vi "BRig_RT_panel_Laser2_v0,90.vi"(7 "input_setValues":bool, 9 "input_dataExp":u16[](array[numeric]), 11 "input_dataLC":u16[](array[numeric])) -> (1 "output_dataExp":u16[](array[numeric]), 3 "output_dataLC":u16[](array[numeric]))   [LabVIEW 2014]
panel:
  in  "LED_baseline":bool
  in  "Laser_power_step":dbl
  in  "Laser_power_max":dbl
  in  "Laser_power_min":dbl
  in  "Laser_Tshutter":u16=2
  in  "Laser_Freq":u16=10
  in  "Laser_Tpeak":u16=2
  in  "Laser_T":u16
  in  "LC_Sel_PostR_Count":u16
  in  "LC_Sel_PostR_Probability":u16
  in  "LC_Sel_PostR_Block":u16(slide) max=2 step=1 scale=0.0..2.0
  in  "LC_Sel_PostR_OnOff":bool
  in  "LC_Sel_PostR_Tdelay":u16
  in  "LC_Cue_PostR_Count":u16
  in  "LC_Cue_PostR_delayOpt":bool
  in  "LC_Cue_PostR_Probability":u16
  in  "LC_Cue_PostR_Block":u16(slide) max=2 step=1 scale=0.0..2.0
  in  "LC_Cue_PostR_OnOff":bool
  in  "LC_Cue_PostR_Tdelay":u16
  in  "LC_ENL_PostR_delayOpt":bool
  in  "LC_ENL_PostR_Count":u16
  in  "LC_ENL_PostR_Probability":u16 max=100 step=1
  in  "LC_ENL_PostR_Block":u16(slide) max=2 step=1 scale=0.0..2.0
  in  "LC_ENL_PostR_OnOff":bool
  in  "LC_ENL_PostR_Tdelay":u16
  in  "LC_Sel_PreR_Count":u16
  in  "LC_Sel_First_Count":u16
  in  "LC_Sel_PreR_Probability":u16
  in  "LC_Sel_PreR_Block":u16(slide) max=2 step=1 scale=0.0..2.0
  in  "LC_Sel_PreR_OnOff":bool
  in  "LC_Sel_First_Probability":u16
  in  "LC_Sel_First_Block":u16(slide) max=2 step=1 scale=0.0..2.0
  in  "LC_Sel_First_OnOff":bool
  in  "LC_Sel_PreR_Tdelay":u16
  in  "LC_Sel_First_Tdelay":u16
  in  "LC_Cue_PreR_Count":u16
  in  "LC_Cue_First_Count":u16
  in  "LC_Cue_PreR_delayOpt":bool
  in  "LC_ENL_PreR_delayOpt":bool
  in  "LC_ENL_PreR_Count":u16
  in  "LC_ENL_First_Count":u16
  in  "LC_Cue_First_delayOpt":bool
  in  "LC_ENL_First_delayOpt":bool
  in  "LC_Wrong_Probability":u16
  in  "LC_Wrong_Trial":u16(slide) max=2 step=1 scale=0.0..2.0
  in  "LC_Wrong_Block":u16(slide) max=2 step=1 scale=0.0..2.0
  in  "LC_Wrong_OnOff":bool
  in  "LC_Reward_Probability":u16
  in  "LC_Reward_Trial":u16(slide) max=2 step=1 scale=0.0..2.0
  in  "LC_Reward_Block":u16(slide) max=2 step=1 scale=0.0..2.0
  in  "LC_Reward_OnOff":bool
  in  "LC_Cue_PreR_Probability":u16
  in  "LC_Cue_PreR_Block":u16(slide) max=2 step=1 scale=0.0..2.0
  in  "LC_Cue_PreR_OnOff":bool
  in  "LC_Cue_First_Probability":u16
  in  "LC_Cue_First_Block":u16(slide) max=2 step=1 scale=0.0..2.0
  in  "LC_Cue_First_OnOff":bool
  in  "LC_ENL_PreR_Probability":u16 max=100 step=1
  in  "LC_ENL_PreR_Block":u16(slide) max=2 step=1 scale=0.0..2.0
  in  "LC_ENL_PreR_OnOff":bool
  in  "LC_ENL_First_Probability":u16 max=100 step=1
  in  "LC_ENL_First_Block":u16(slide) max=2 step=1 scale=0.0..2.0
  in  "LC_Wrong_Tdelay":u16
  in  "LC_Cue_PreR_Tdelay":u16
  in  "LC_ENL_PreR_Tdelay":u16
  in  "LC_Reward_Tdelay":u16
  in  "LC_Cue_First_Tdelay":u16
  in  "LC_ENL_First_Tdelay":u16
  in  "LC_ENL_First_OnOff":bool
  # "Laser2 Control\n                               On/Off      Block        Probability [%]   Delay [ms]                              Count"
  # "Enforced\nNonLick"
  # "from end"
  # "First\nTrial"
  # "from start"
  # "from end"
  # "PreReward\nTrials"
  # "from start"
  # "from end"
  # "PostReward\nTrials"
  # "from start"
  # "Cue"
  # "from end"
  # "First\nTrial"
  # "from start"
  # "from end"
  # "PreReward\nTrials"
  # "from start"
  # "from end"
  # "PreReward\nTrials"
  # "from start"
  # "Selection"
  # "from start"
  # "First\nTrial"
  # "from start"
  # "PreReward\nTrials"
  # "from start"
  # "PostReward\nTrials"
  # "Laser2 Parameters"
  # "Laser2 Response\n           On/Off      Block           Trial     Probability %  Delay [ms]"
  # "Frequency\n[Hz]"
  # "Selection\nReward"
  # "Timing [ms]\n Duration     Peak Width   Shutter"
  # "Selection\nWrong"
  # "Laser Power [V]\nMin          Max              Step"
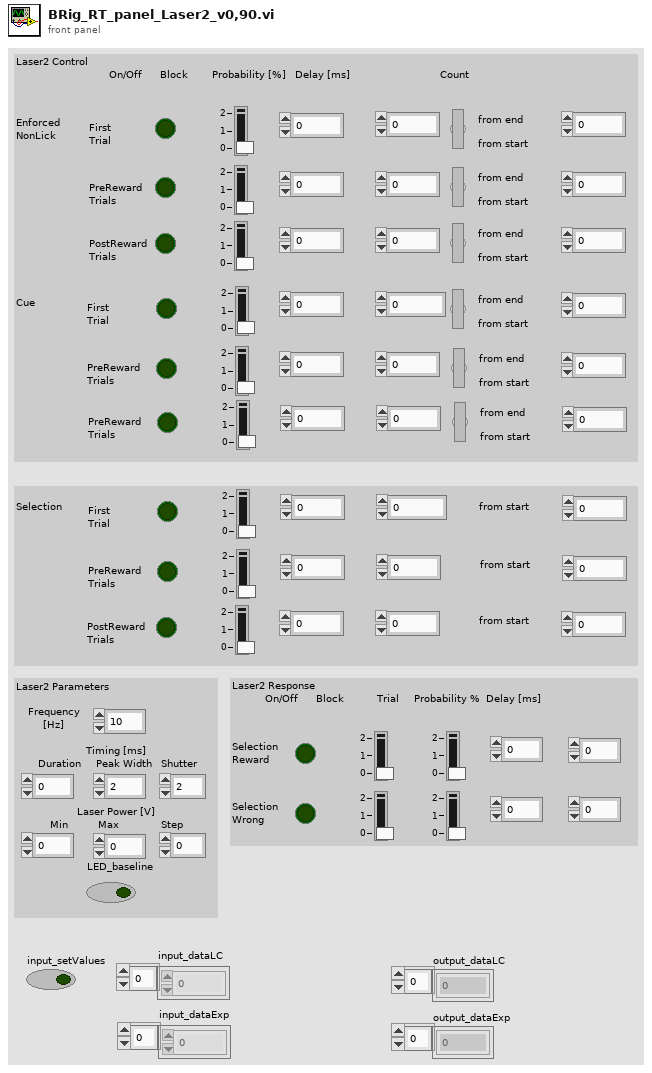
[diagram p1: front panel]
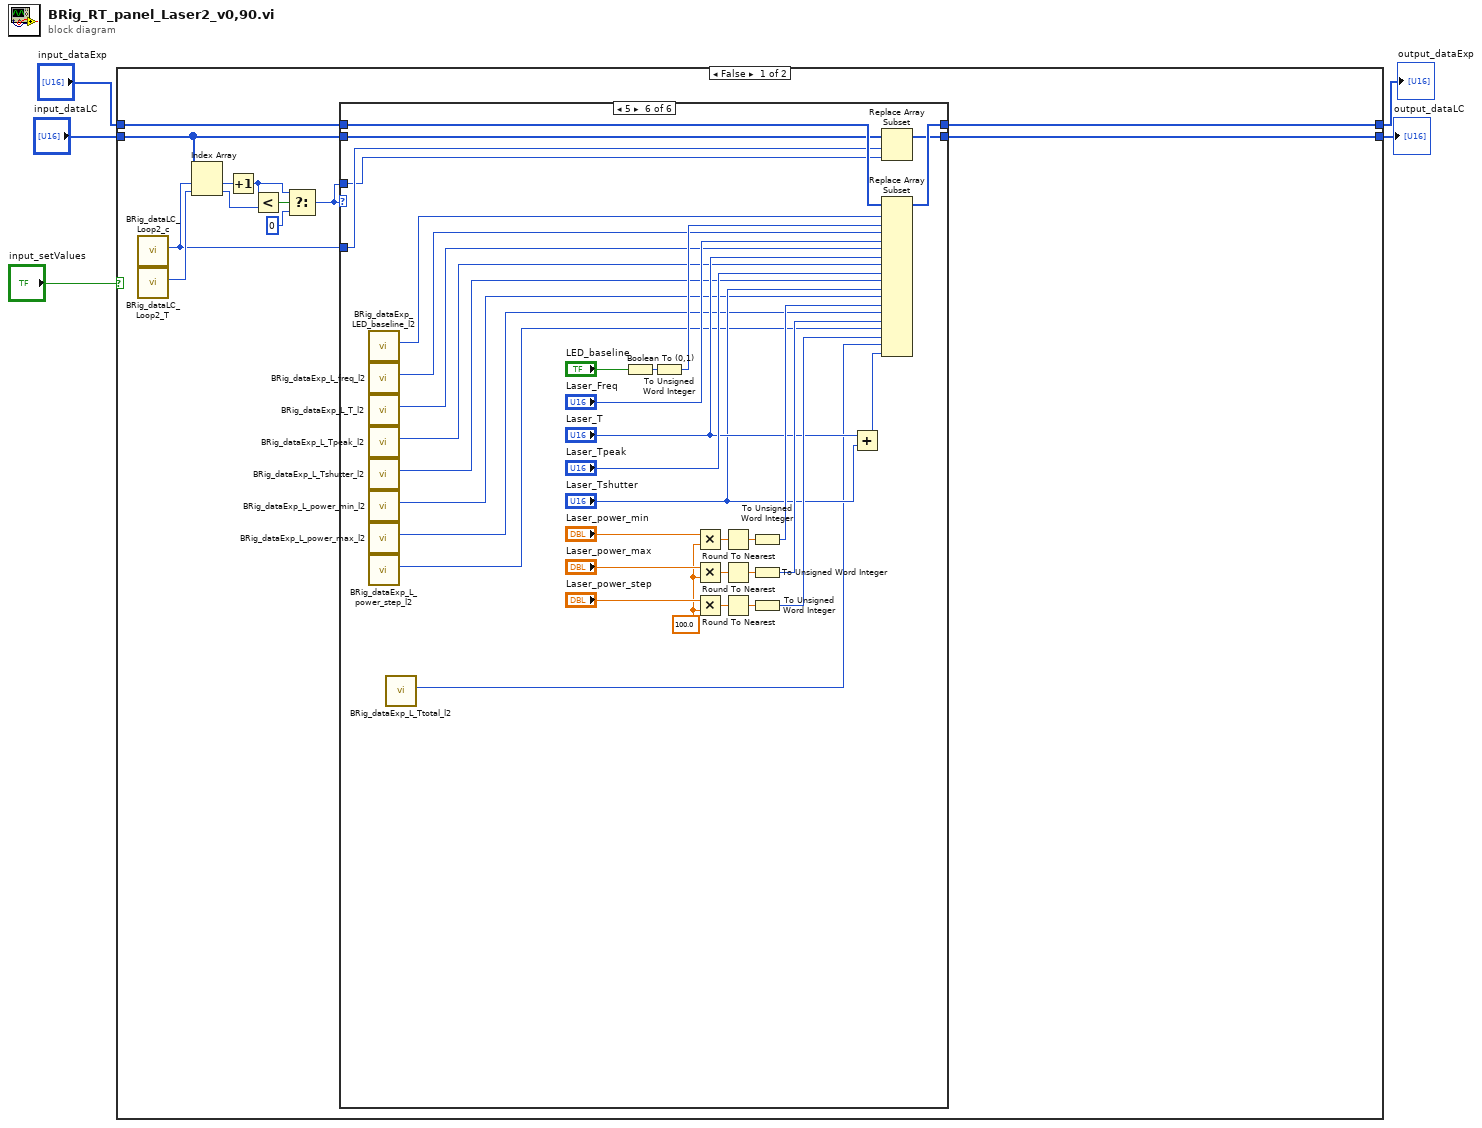
[diagram p0: block diagram]
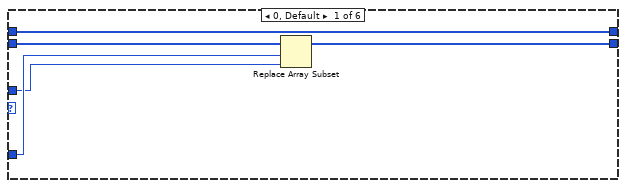
[diagram p2: hidden frame]
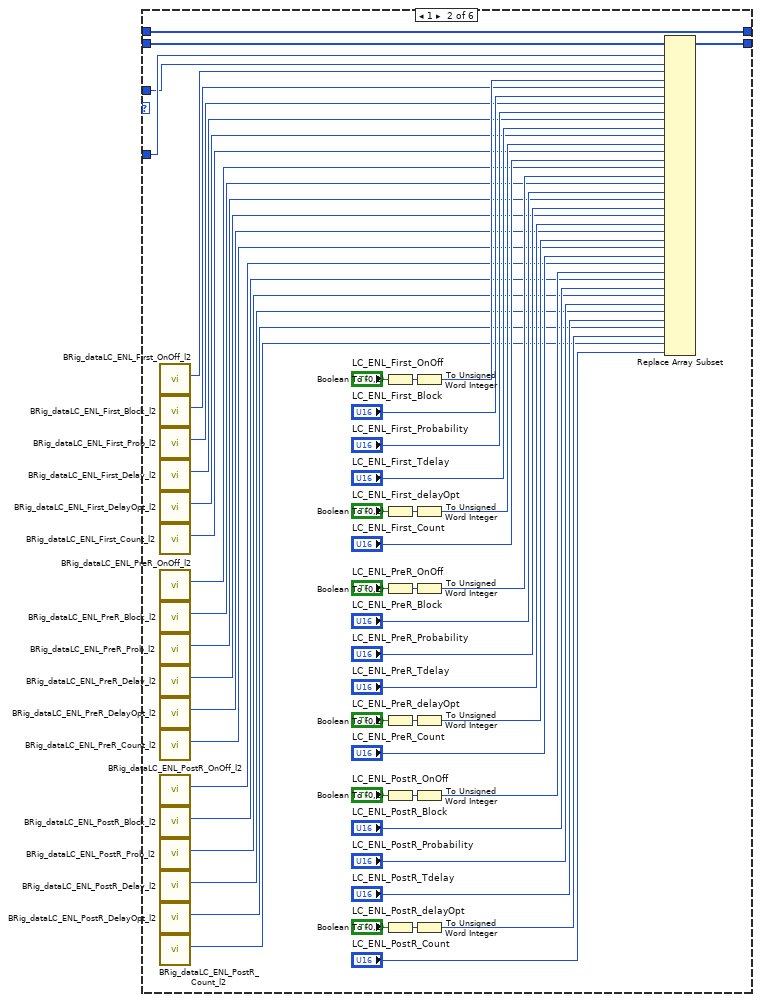
[diagram p3: hidden frame]
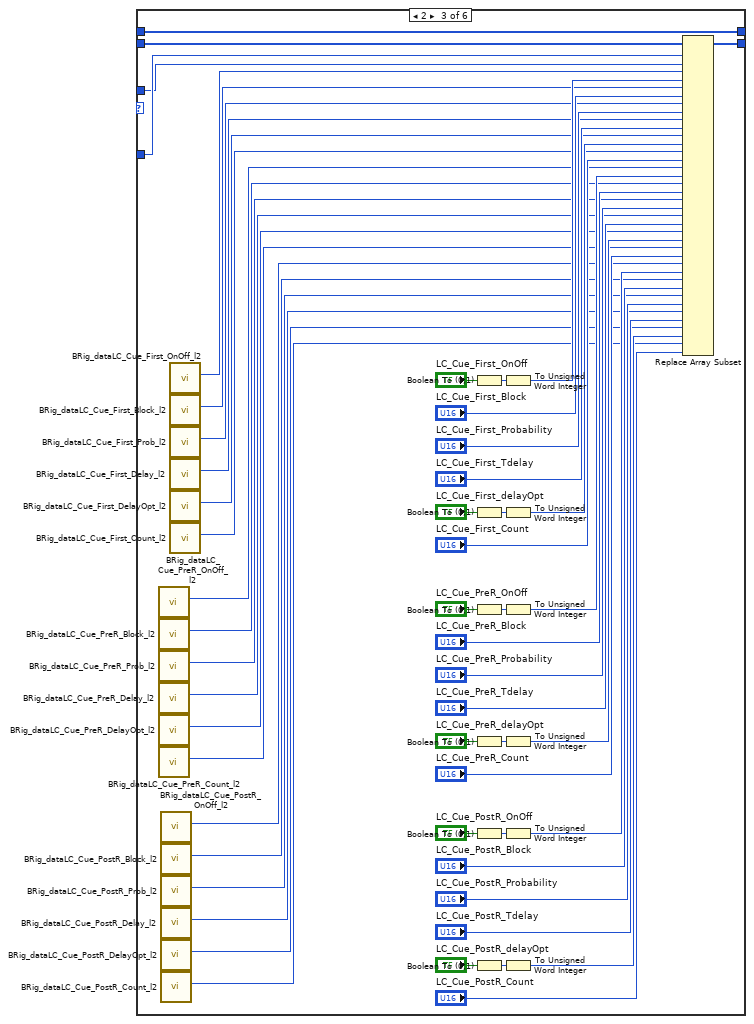
[diagram p4: hidden frame]
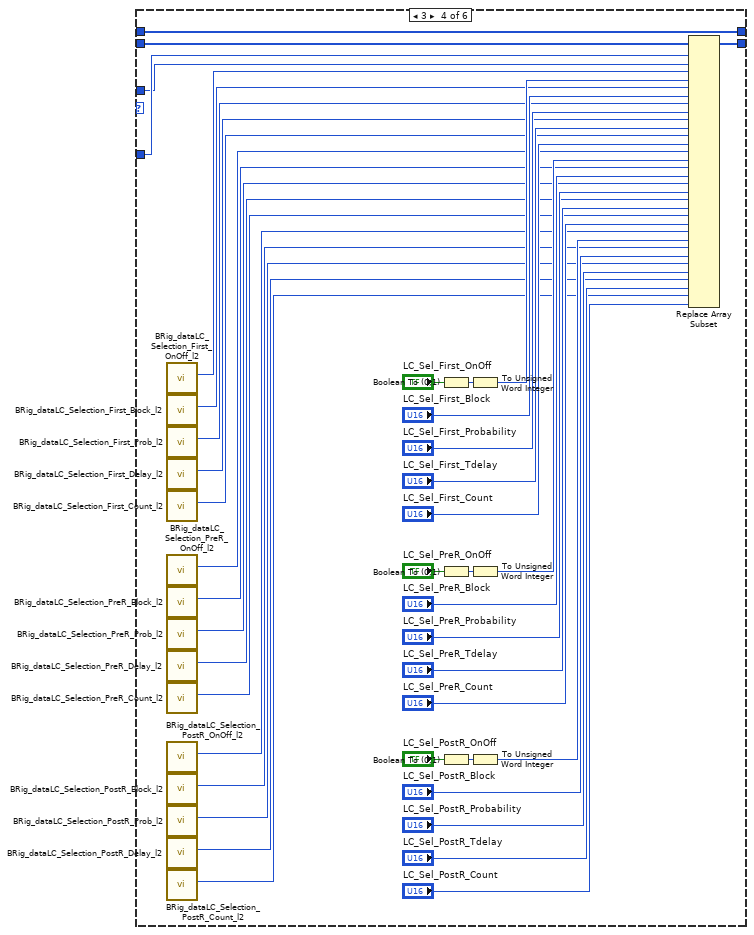
[diagram p5: hidden frame]
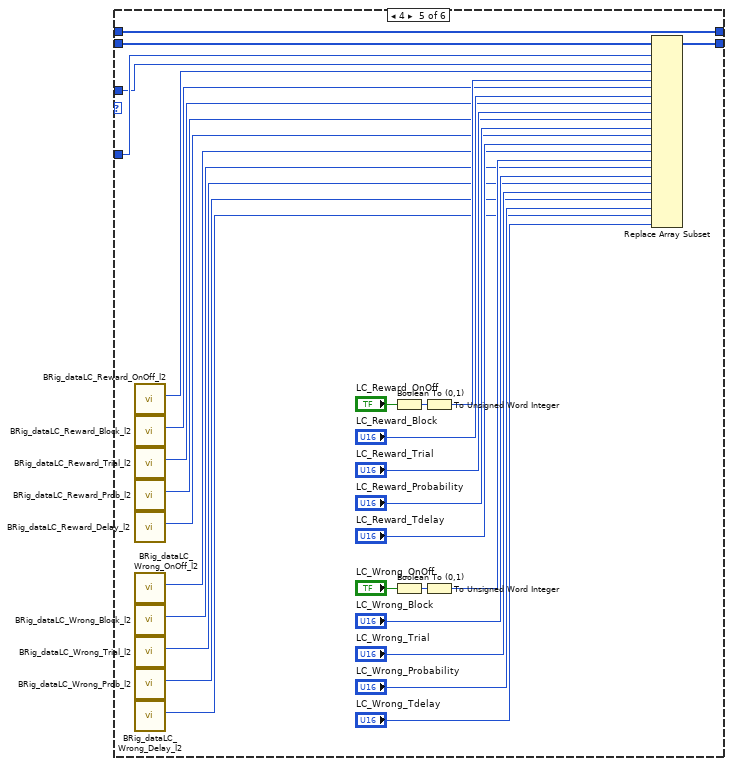
[diagram p6: hidden frame]
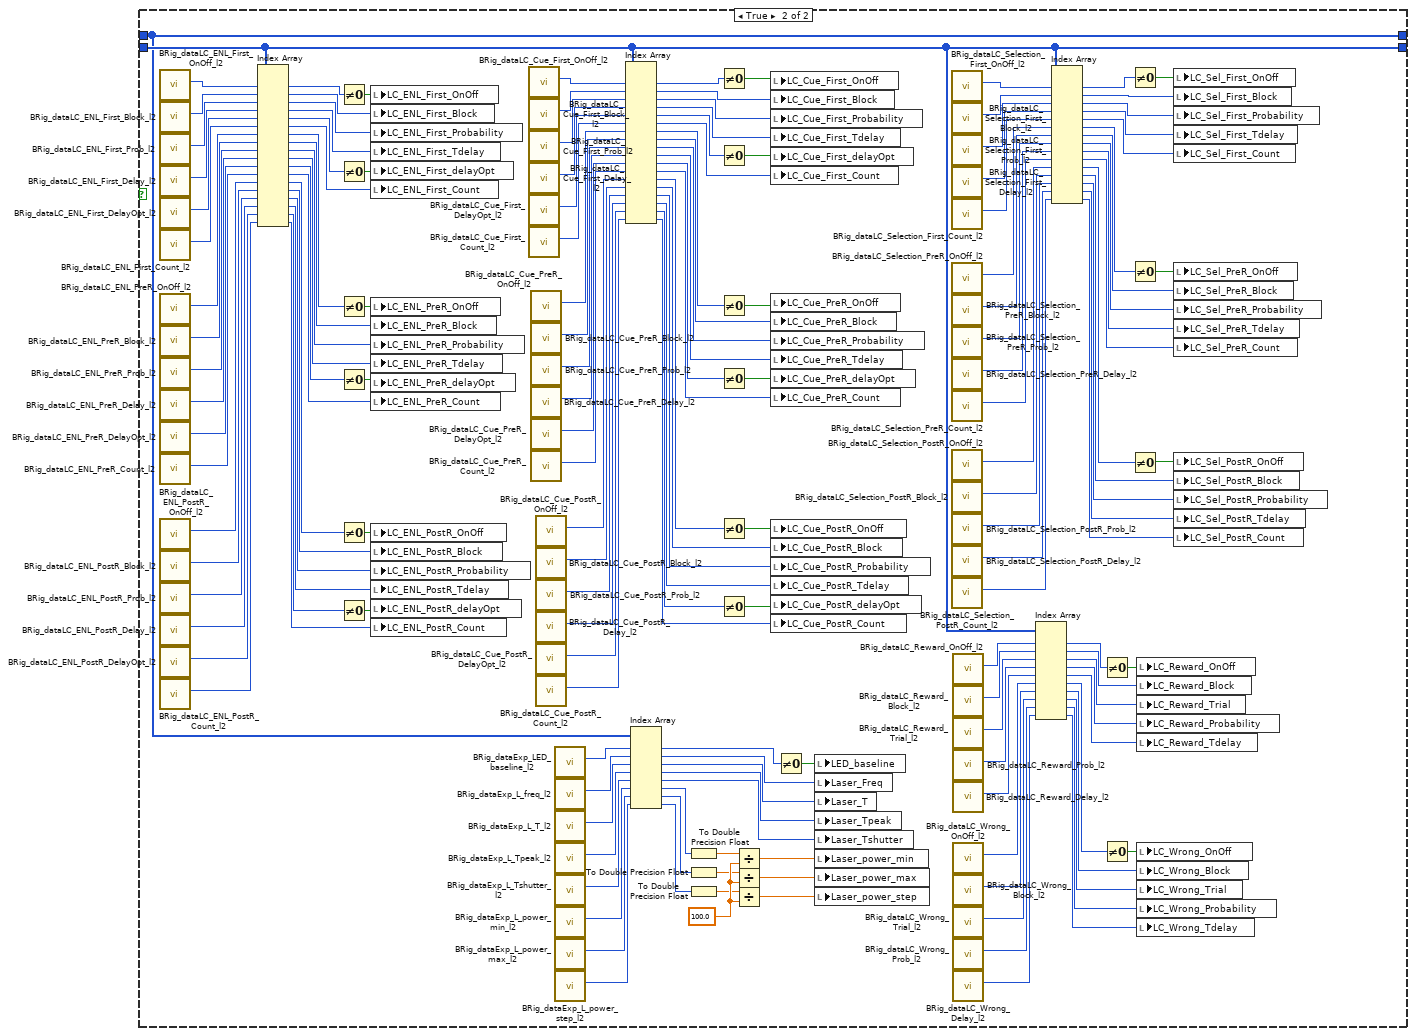
[diagram p7: hidden frame]
diagram:
  n1 = case shown="False" "input_setValues" {
    tunnel: "input_dataLC" -> [w17 w321]
    tunnel: [w11 w321] -> w4
    tunnel: "input_dataExp" -> [w7 w235]
    tunnel: [w6 w235] -> w1
    frame False {
      n2 = call "BRig_dataLC_Loop2_c.vi"() -> ("output_Loop2_c"=w8:i32)  [unwired: 11 in]
      n3 = call "BRig_dataLC_Loop2_T.vi"() -> ("output_Loop2_T"=w9:i32)  [unwired: 11 in]
      n4 = Index Array(array=w17, index #1=w8, index #2=w9) -> (element #1=w16:u16, element #2=w15:u16)
      n5 = Increment(x=w16) -> (x+1=w12:u16)
      n6 = Less?(x=w12, y=w15) -> (x < y?=w14:bool)
      n7 = Select(t=w12, s=w14, f=u16 0) -> (s? t:f=w10:u16)
      n8 = case shown="5" w10 {
        tunnel: w17 -> [w22 w75 w128 w169 w198 w202]
        tunnel: w8 -> [w20 w43 w96 w146 w182 w200]
        tunnel: w10 -> [w19 w42 w95 w145 w181 w199]
        tunnel: [w21 w74 w127 w168 w197 w201] -> w11
        tunnel: w7 -> [w18 w23 w76 w129 w170 w204]
        tunnel: [w18 w23 w76 w129 w170 w203] -> w6
        frame 0, Default {
          n9 = Replace Array Subset(array=w22, new element=w19, index=w20) -> (w21:u16[])
        }
        frame 1 {
          n10 = call "BRig_dataLC_ENL_First_OnOff_l2.vi"() -> ("output_ENL_First_OnOff_l2"=w24:i32)  [unwired: 11 in]
          n11 = call "BRig_dataLC_ENL_First_Block_l2.vi"() -> ("output_ENL_First_Block_l2"=w25:i32)  [unwired: 11 in]
          n12 = call "BRig_dataLC_ENL_First_Prob_l2.vi"() -> ("output_ENL_First_Prob_l2"=w26:i32)  [unwired: 11 in]
          n13 = call "BRig_dataLC_ENL_First_Delay_l2.vi"() -> ("output_ENL_First_Delay_l2"=w27:i32)  [unwired: 11 in]
          n14 = call "BRig_dataLC_ENL_First_DelayOpt_l2.vi"() -> ("output_ENL_First_DelayOpt_l2"=w28:i32)  [unwired: 11 in]
          n15 = call "BRig_dataLC_ENL_First_Count_l2.vi"() -> ("output_ENL_First_Count_l2"=w39:i32)  [unwired: 11 in]
          n16 = call "BRig_dataLC_ENL_PreR_OnOff_l2.vi"() -> ("output_ENL_PreR_OnOff_l2"=w29:i32)  [unwired: 11 in]
          n17 = call "BRig_dataLC_ENL_PreR_Block_l2.vi"() -> ("output_ENL_PreR_Block_l2"=w31:i32)  [unwired: 11 in]
          n18 = call "BRig_dataLC_ENL_PreR_Prob_l2.vi"() -> ("output_ENL_PreR_Prob_l2"=w30:i32)  [unwired: 11 in]
          n19 = call "BRig_dataLC_ENL_PreR_Delay_l2.vi"() -> ("output_ENL_PreR_Delay_l2"=w32:i32)  [unwired: 11 in]
          n20 = call "BRig_dataLC_ENL_PreR_DelayOpt_l2.vi"() -> ("output_ENL_PreR_DelayOpt_l2"=w33:i32)  [unwired: 11 in]
          n21 = call "BRig_dataLC_ENL_PreR_Count_l2.vi"() -> ("output_ENL_PreR_Count_l2"=w40:i32)  [unwired: 11 in]
          n22 = call "BRig_dataLC_ENL_PostR_OnOff_l2.vi"() -> ("output_ENL_PostR_OnOff_l2"=w34:i32)  [unwired: 11 in]
          n23 = call "BRig_dataLC_ENL_PostR_Block_l2.vi"() -> ("output_ENL_PostR_Block_l2"=w35:i32)  [unwired: 11 in]
          n24 = call "BRig_dataLC_ENL_PostR_Prob_l2.vi"() -> ("output_ENL_PostR_Prob_l2"=w36:i32)  [unwired: 11 in]
          n25 = call "BRig_dataLC_ENL_PostR_Delay_l2.vi"() -> ("output_ENL_PostR_Delay_l2"=w37:i32)  [unwired: 11 in]
          n26 = call "BRig_dataLC_ENL_PostR_DelayOpt_l2.vi"() -> ("output_ENL_PostR_DelayOpt_l2"=w38:i32)  [unwired: 11 in]
          n27 = call "BRig_dataLC_ENL_PostR_Count_l2.vi"() -> ("output_ENL_PostR_Count_l2"=w41:i32)  [unwired: 11 in]
          n28 = Boolean To (0,1)(Boolean="LC_ENL_First_OnOff") -> (0, 1=w72:i16)
          n29 = Boolean To (0,1)(Boolean="LC_ENL_First_delayOpt") -> (0, 1=w71:i16)
          n30 = Boolean To (0,1)(Boolean="LC_ENL_PreR_OnOff") -> (0, 1=w69:i16)
          n31 = Boolean To (0,1)(Boolean="LC_ENL_PreR_delayOpt") -> (0, 1=w67:i16)
          n32 = Boolean To (0,1)(Boolean="LC_ENL_PostR_OnOff") -> (0, 1=w65:i16)
          n33 = Boolean To (0,1)(Boolean="LC_ENL_PostR_delayOpt") -> (0, 1=w63:i16)
          n34 = To Unsigned Word Integer(number=w72) -> (unsigned 16bit integer=w61:u16)
          n35 = To Unsigned Word Integer(number=w71) -> (unsigned 16bit integer=w57:u16)
          n36 = To Unsigned Word Integer(number=w69) -> (unsigned 16bit integer=w55:u16)
          n37 = To Unsigned Word Integer(number=w67) -> (unsigned 16bit integer=w51:u16)
          n38 = To Unsigned Word Integer(number=w65) -> (unsigned 16bit integer=w49:u16)
          n39 = To Unsigned Word Integer(number=w63) -> (unsigned 16bit integer=w45:u16)
          n40 = Replace Array Subset(array=w75, new element #1=w42, index #1=w43, new element #2=w61, index #2=w24, new element #3="LC_ENL_First_Block", index #3=w25, new element #4="LC_ENL_First_Probability", index #4=w26, new element #5="LC_ENL_First_Tdelay", index #5=w27, new element #6=w57, index #6=w28, new element #7="LC_ENL_First_Count", index #7=w39, new element #8=w55, index #8=w29, new element #9="LC_ENL_PreR_Block", index #9=w31, new element #10="LC_ENL_PreR_Probability", index #10=w30, new element #11="LC_ENL_PreR_Tdelay", index #11=w32, new element #12=w51, index #12=w33, new element #13="LC_ENL_PreR_Count", index #13=w40, new element #14=w49, index #14=w34, new element #15="LC_ENL_PostR_Block", index #15=w35, new element #16="LC_ENL_PostR_Probability", index #16=w36, new element #17="LC_ENL_PostR_Tdelay", index #17=w37, new element #18=w45, index #18=w38, new element #19="LC_ENL_PostR_Count", index #19=w41) -> (w74:u16[])
        }
        frame 2 {
          n41 = call "BRig_dataLC_Cue_PreR_OnOff_l2.vi"() -> ("output_Cue_PreR_OnOff_l2"=w83:i32)  [unwired: 11 in]
          n42 = call "BRig_dataLC_Cue_PreR_Block_l2.vi"() -> ("output_Cue_PreR_Block_l2"=w84:i32)  [unwired: 11 in]
          n43 = call "BRig_dataLC_Cue_PreR_Prob_l2.vi"() -> ("output_Cue_PreR_Prob_l2"=w85:i32)  [unwired: 11 in]
          n44 = call "BRig_dataLC_Cue_PreR_Delay_l2.vi"() -> ("output_Cue_PreR_Delay_l2"=w86:i32)  [unwired: 11 in]
          n45 = call "BRig_dataLC_Cue_PreR_DelayOpt_l2.vi"() -> ("output_Cue_PreR_DelayOpt_l2"=w87:i32)  [unwired: 11 in]
          n46 = call "BRig_dataLC_Cue_PreR_Count_l2.vi"() -> ("output_Cue_PreR_Count_l2"=w88:i32)  [unwired: 11 in]
          n47 = call "BRig_dataLC_Cue_PostR_OnOff_l2.vi"() -> ("output_Cue_PostR_OnOff_l2"=w82:i32)  [unwired: 11 in]
          n48 = call "BRig_dataLC_Cue_PostR_Block_l2.vi"() -> ("output_Cue_PostR_Block_l2"=w77:i32)  [unwired: 11 in]
          n49 = call "BRig_dataLC_Cue_PostR_Prob_l2.vi"() -> ("output_Cue_PostR_Prob_l2"=w78:i32)  [unwired: 11 in]
          n50 = call "BRig_dataLC_Cue_PostR_Delay_l2.vi"() -> ("output_Cue_PostR_Delay_l2"=w79:i32)  [unwired: 11 in]
          n51 = call "BRig_dataLC_Cue_PostR_DelayOpt_l2.vi"() -> ("output_Cue_PostR_DelayOpt_l2"=w80:i32)  [unwired: 11 in]
          n52 = call "BRig_dataLC_Cue_PostR_Count_l2.vi"() -> ("output_Cue_PostR_Count_l2"=w81:i32)  [unwired: 11 in]
          n53 = call "BRig_dataLC_Cue_First_OnOff_l2.vi"() -> ("output_Cue_First_OnOff_l2"=w89:i32)  [unwired: 11 in]
          n54 = call "BRig_dataLC_Cue_First_Block_l2.vi"() -> ("output_Cue_First_Block_l2"=w90:i32)  [unwired: 11 in]
          n55 = call "BRig_dataLC_Cue_First_Prob_l2.vi"() -> ("output_Cue_First_Prob_l2"=w91:i32)  [unwired: 11 in]
          n56 = call "BRig_dataLC_Cue_First_Delay_l2.vi"() -> ("output_Cue_First_Delay_l2"=w92:i32)  [unwired: 11 in]
          n57 = call "BRig_dataLC_Cue_First_DelayOpt_l2.vi"() -> ("output_Cue_First_DelayOpt_l2"=w93:i32)  [unwired: 11 in]
          n58 = call "BRig_dataLC_Cue_First_Count_l2.vi"() -> ("output_Cue_First_Count_l2"=w94:i32)  [unwired: 11 in]
          n59 = Boolean To (0,1)(Boolean="LC_Cue_First_OnOff") -> (0, 1=w120:i16)
          n60 = Boolean To (0,1)(Boolean="LC_Cue_First_delayOpt") -> (0, 1=w119:i16)
          n61 = Boolean To (0,1)(Boolean="LC_Cue_PreR_OnOff") -> (0, 1=w118:i16)
          n62 = Boolean To (0,1)(Boolean="LC_Cue_PreR_delayOpt") -> (0, 1=w117:i16)
          n63 = Boolean To (0,1)(Boolean="LC_Cue_PostR_OnOff") -> (0, 1=w116:i16)
          n64 = Boolean To (0,1)(Boolean="LC_Cue_PostR_delayOpt") -> (0, 1=w115:i16)
          n65 = To Unsigned Word Integer(number=w120) -> (unsigned 16bit integer=w114:u16)
          n66 = To Unsigned Word Integer(number=w119) -> (unsigned 16bit integer=w110:u16)
          n67 = To Unsigned Word Integer(number=w118) -> (unsigned 16bit integer=w108:u16)
          n68 = To Unsigned Word Integer(number=w117) -> (unsigned 16bit integer=w104:u16)
          n69 = To Unsigned Word Integer(number=w116) -> (unsigned 16bit integer=w102:u16)
          n70 = To Unsigned Word Integer(number=w115) -> (unsigned 16bit integer=w98:u16)
          n71 = Replace Array Subset(array=w128, new element #1=w95, index #1=w96, new element #2=w114, index #2=w89, new element #3="LC_Cue_First_Block", index #3=w90, new element #4="LC_Cue_First_Probability", index #4=w91, new element #5="LC_Cue_First_Tdelay", index #5=w92, new element #6=w110, index #6=w93, new element #7="LC_Cue_First_Count", index #7=w94, new element #8=w108, index #8=w83, new element #9="LC_Cue_PreR_Block", index #9=w84, new element #10="LC_Cue_PreR_Probability", index #10=w85, new element #11="LC_Cue_PreR_Tdelay", index #11=w86, new element #12=w104, index #12=w87, new element #13="LC_Cue_PreR_Count", index #13=w88, new element #14=w102, index #14=w82, new element #15="LC_Cue_PostR_Block", index #15=w77, new element #16="LC_Cue_PostR_Probability", index #16=w78, new element #17="LC_Cue_PostR_Tdelay", index #17=w79, new element #18=w98, index #18=w80, new element #19="LC_Cue_PostR_Count", index #19=w81) -> (w127:u16[])
        }
        frame 3 {
          n72 = call "BRig_dataLC_Selection_First_OnOff_l2.vi"() -> ("output_Selection_First_OnOff_l2"=w130:i32)  [unwired: 11 in]
          n73 = call "BRig_dataLC_Selection_First_Block_l2.vi"() -> ("output_Selection_First_Block_l2"=w131:i32)  [unwired: 11 in]
          n74 = call "BRig_dataLC_Selection_First_Prob_l2.vi"() -> ("output_Selection_First_Prob_l2"=w132:i32)  [unwired: 11 in]
          n75 = call "BRig_dataLC_Selection_First_Delay_l2.vi"() -> ("output_Selection_First_Delay_l2"=w133:i32)  [unwired: 11 in]
          n76 = call "BRig_dataLC_Selection_First_Count_l2.vi"() -> ("output_Selection_First_Count_l2"=w134:i32)  [unwired: 11 in]
          n77 = call "BRig_dataLC_Selection_PreR_OnOff_l2.vi"() -> ("output_Selection_PreR_OnOff_l2"=w135:i32)  [unwired: 11 in]
          n78 = call "BRig_dataLC_Selection_PreR_Block_l2.vi"() -> ("output_Selection_PreR_Block_l2"=w136:i32)  [unwired: 11 in]
          n79 = call "BRig_dataLC_Selection_PreR_Prob_l2.vi"() -> ("output_Selection_PreR_Prob_l2"=w137:i32)  [unwired: 11 in]
          n80 = call "BRig_dataLC_Selection_PreR_Delay_l2.vi"() -> ("output_Selection_PreR_Delay_l2"=w138:i32)  [unwired: 11 in]
          n81 = call "BRig_dataLC_Selection_PreR_Count_l2.vi"() -> ("output_Selection_PreR_Count_l2"=w139:i32)  [unwired: 11 in]
          n82 = call "BRig_dataLC_Selection_PostR_OnOff_l2.vi"() -> ("output_Selection_PostR_OnOff_l2"=w140:i32)  [unwired: 11 in]
          n83 = call "BRig_dataLC_Selection_PostR_Block_l2.vi"() -> ("output_Selection_PostR_Block_l2"=w141:i32)  [unwired: 11 in]
          n84 = call "BRig_dataLC_Selection_PostR_Prob_l2.vi"() -> ("output_Selection_PostR_Prob_l2"=w142:i32)  [unwired: 11 in]
          n85 = call "BRig_dataLC_Selection_PostR_Delay_l2.vi"() -> ("output_Selection_PostR_Delay_l2"=w143:i32)  [unwired: 11 in]
          n86 = call "BRig_dataLC_Selection_PostR_Count_l2.vi"() -> ("output_Selection_PostR_Count_l2"=w144:i32)  [unwired: 11 in]
          n87 = Boolean To (0,1)(Boolean="LC_Sel_First_OnOff") -> (0, 1=w164:i16)
          n88 = Boolean To (0,1)(Boolean="LC_Sel_PreR_OnOff") -> (0, 1=w163:i16)
          n89 = Boolean To (0,1)(Boolean="LC_Sel_PostR_OnOff") -> (0, 1=w162:i16)
          n90 = To Unsigned Word Integer(number=w164) -> (unsigned 16bit integer=w161:u16)
          n91 = To Unsigned Word Integer(number=w163) -> (unsigned 16bit integer=w156:u16)
          n92 = To Unsigned Word Integer(number=w162) -> (unsigned 16bit integer=w151:u16)
          n93 = Replace Array Subset(array=w169, new element #1=w145, index #1=w146, new element #2=w161, index #2=w130, new element #3="LC_Sel_First_Block", index #3=w131, new element #4="LC_Sel_First_Probability", index #4=w132, new element #5="LC_Sel_First_Tdelay", index #5=w133, new element #6="LC_Sel_First_Count", index #6=w134, new element #7=w156, index #7=w135, new element #8="LC_Sel_PreR_Block", index #8=w136, new element #9="LC_Sel_PreR_Probability", index #9=w137, new element #10="LC_Sel_PreR_Tdelay", index #10=w138, new element #11="LC_Sel_PreR_Count", index #11=w139, new element #12=w151, index #12=w140, new element #13="LC_Sel_PostR_Block", index #13=w141, new element #14="LC_Sel_PostR_Probability", index #14=w142, new element #15="LC_Sel_PostR_Tdelay", index #15=w143, new element #16="LC_Sel_PostR_Count", index #16=w144) -> (w168:u16[])
        }
        frame 4 {
          n94 = call "BRig_dataLC_Reward_OnOff_l2.vi"() -> ("output_Reward_OnOff_l2"=w171:i32)  [unwired: 11 in]
          n95 = call "BRig_dataLC_Reward_Block_l2.vi"() -> ("output_Reward_Block_l2"=w172:i32)  [unwired: 11 in]
          n96 = call "BRig_dataLC_Reward_Trial_l2.vi"() -> ("output_Reward_Trial_l2"=w173:i32)  [unwired: 11 in]
          n97 = call "BRig_dataLC_Reward_Prob_l2.vi"() -> ("output_Reward_Prob_l2"=w174:i32)  [unwired: 11 in]
          n98 = call "BRig_dataLC_Reward_Delay_l2.vi"() -> ("output_Reward_Delay_l2"=w175:i32)  [unwired: 11 in]
          n99 = call "BRig_dataLC_Wrong_OnOff_l2.vi"() -> ("output_Wrong_OnOff_l2"=w176:i32)  [unwired: 11 in]
          n100 = call "BRig_dataLC_Wrong_Block_l2.vi"() -> ("output_Wrong_Block_l2"=w177:i32)  [unwired: 11 in]
          n101 = call "BRig_dataLC_Wrong_Trial_l2.vi"() -> ("output_Wrong_Trial_l2"=w178:i32)  [unwired: 11 in]
          n102 = call "BRig_dataLC_Wrong_Prob_l2.vi"() -> ("output_Wrong_Prob_l2"=w179:i32)  [unwired: 11 in]
          n103 = call "BRig_dataLC_Wrong_Delay_l2.vi"() -> ("output_Wrong_Delay_l2"=w180:i32)  [unwired: 11 in]
          n104 = Boolean To (0,1)(Boolean="LC_Reward_OnOff") -> (0, 1=w194:i16)
          n105 = Boolean To (0,1)(Boolean="LC_Wrong_OnOff") -> (0, 1=w193:i16)
          n106 = To Unsigned Word Integer(number=w194) -> (unsigned 16bit integer=w192:u16)
          n107 = To Unsigned Word Integer(number=w193) -> (unsigned 16bit integer=w187:u16)
          n108 = Replace Array Subset(array=w198, new element #1=w181, index #1=w182, new element #2=w192, index #2=w171, new element #3="LC_Reward_Block", index #3=w172, new element #4="LC_Reward_Trial", index #4=w173, new element #5="LC_Reward_Probability", index #5=w174, new element #6="LC_Reward_Tdelay", index #6=w175, new element #7=w187, index #7=w176, new element #8="LC_Wrong_Block", index #8=w177, new element #9="LC_Wrong_Trial", index #9=w178, new element #10="LC_Wrong_Probability", index #10=w179, new element #11="LC_Wrong_Tdelay", index #11=w180) -> (w197:u16[])
        }
        frame 5 {
          w222 = 100.0 ("y")
          n109 = call "BRig_dataExp_LED_baseline_l2.vi"() -> ("output_LED_baseline_l2"=w212:i32)  [unwired: 11 in]
          n110 = call "BRig_dataExp_L_freq_l2.vi"() -> ("output_L_freq_l2"=w211:i32)  [unwired: 11 in]
          n111 = call "BRig_dataExp_L_T_l2.vi"() -> ("output_L_T_l2"=w210:i32)  [unwired: 11 in]
          n112 = call "BRig_dataExp_L_Tpeak_l2.vi"() -> ("output_L_Tpeak_l2"=w209:i32)  [unwired: 11 in]
          n113 = call "BRig_dataExp_L_Tshutter_l2.vi"() -> ("output_L_Tshutter_l2"=w208:i32)  [unwired: 11 in]
          n114 = call "BRig_dataExp_L_power_min_l2.vi"() -> ("output_L_power_min_l2"=w207:i32)  [unwired: 11 in]
          n115 = call "BRig_dataExp_L_power_max_l2.vi"() -> ("output_L_power_max_l2"=w206:i32)  [unwired: 11 in]
          n116 = call "BRig_dataExp_L_power_step_l2.vi"() -> ("output_L_power_step_l2"=w205:i32)  [unwired: 11 in]
          n117 = call "BRig_dataExp_L_Ttotal_l2.vi"() -> ("output_L_Ttotal_l2"=w213:i32)  [unwired: 11 in]
          n118 = Boolean To (0,1)(Boolean="LED_baseline") -> (0, 1=w234:i16)
          n119 = To Unsigned Word Integer(number=w234) -> (unsigned 16bit integer=w232:u16)
          n120 = Multiply(x="Laser_power_min", y=w222) -> (x*y=w226:dbl)
          n121 = Multiply(x="Laser_power_max", y=w222) -> (x*y=w228:dbl)
          n122 = Multiply(x="Laser_power_step", y=w222) -> (x*y=w231:dbl)
          n123 = Round To Nearest(number=w226) -> (nearest integer value=w225:dbl)
          n124 = Round To Nearest(number=w228) -> (nearest integer value=w227:dbl)
          n125 = Round To Nearest(number=w231) -> (nearest integer value=w230:dbl)
          n126 = To Unsigned Word Integer(number=w225) -> (unsigned 16bit integer=w219:u16)
          n127 = To Unsigned Word Integer(number=w227) -> (unsigned 16bit integer=w220:u16)
          n128 = To Unsigned Word Integer(number=w230) -> (unsigned 16bit integer=w221:u16)
          n129 = Add(x="Laser_T", y="Laser_Tshutter") -> (x+y=w214:u16)
          n130 = Replace Array Subset(array=w202, new element=w199, index=w200) -> (w201:u16[])
          n131 = Replace Array Subset(array=w204, new element #1=w232, index #1=w212, new element #2="Laser_Freq", index #2=w211, new element #3="Laser_T", index #3=w210, new element #4="Laser_Tpeak", index #4=w209, new element #5="Laser_Tshutter", index #5=w208, new element #6=w219, index #6=w207, new element #7=w220, index #7=w206, new element #8=w221, index #8=w205, new element #9=w214, index #9=w213) -> (w203:u16[])
        }
      }
    }
    frame True {
      w307 = 100.0 ("y")
      n132 = call "BRig_dataLC_ENL_First_OnOff_l2.vi"() -> ("output_ENL_First_OnOff_l2"=w287:i32)  [unwired: 11 in]
      n133 = call "BRig_dataLC_ENL_First_Block_l2.vi"() -> ("output_ENL_First_Block_l2"=w288:i32)  [unwired: 11 in]
      n134 = call "BRig_dataLC_ENL_First_Prob_l2.vi"() -> ("output_ENL_First_Prob_l2"=w289:i32)  [unwired: 11 in]
      n135 = call "BRig_dataLC_ENL_First_Delay_l2.vi"() -> ("output_ENL_First_Delay_l2"=w290:i32)  [unwired: 11 in]
      n136 = call "BRig_dataLC_ENL_First_DelayOpt_l2.vi"() -> ("output_ENL_First_DelayOpt_l2"=w291:i32)  [unwired: 11 in]
      n137 = call "BRig_dataLC_ENL_First_Count_l2.vi"() -> ("output_ENL_First_Count_l2"=w302:i32)  [unwired: 11 in]
      n138 = call "BRig_dataLC_ENL_PreR_OnOff_l2.vi"() -> ("output_ENL_PreR_OnOff_l2"=w292:i32)  [unwired: 11 in]
      n139 = call "BRig_dataLC_ENL_PreR_Block_l2.vi"() -> ("output_ENL_PreR_Block_l2"=w293:i32)  [unwired: 11 in]
      n140 = call "BRig_dataLC_ENL_PreR_Prob_l2.vi"() -> ("output_ENL_PreR_Prob_l2"=w294:i32)  [unwired: 11 in]
      n141 = call "BRig_dataLC_ENL_PreR_Delay_l2.vi"() -> ("output_ENL_PreR_Delay_l2"=w295:i32)  [unwired: 11 in]
      n142 = call "BRig_dataLC_ENL_PreR_DelayOpt_l2.vi"() -> ("output_ENL_PreR_DelayOpt_l2"=w296:i32)  [unwired: 11 in]
      n143 = call "BRig_dataLC_ENL_PreR_Count_l2.vi"() -> ("output_ENL_PreR_Count_l2"=w303:i32)  [unwired: 11 in]
      n144 = call "BRig_dataLC_ENL_PostR_OnOff_l2.vi"() -> ("output_ENL_PostR_OnOff_l2"=w297:i32)  [unwired: 11 in]
      n145 = call "BRig_dataLC_ENL_PostR_Block_l2.vi"() -> ("output_ENL_PostR_Block_l2"=w298:i32)  [unwired: 11 in]
      n146 = call "BRig_dataLC_ENL_PostR_Prob_l2.vi"() -> ("output_ENL_PostR_Prob_l2"=w299:i32)  [unwired: 11 in]
      n147 = call "BRig_dataLC_ENL_PostR_Delay_l2.vi"() -> ("output_ENL_PostR_Delay_l2"=w300:i32)  [unwired: 11 in]
      n148 = call "BRig_dataLC_ENL_PostR_DelayOpt_l2.vi"() -> ("output_ENL_PostR_DelayOpt_l2"=w301:i32)  [unwired: 11 in]
      n149 = call "BRig_dataLC_ENL_PostR_Count_l2.vi"() -> ("output_ENL_PostR_Count_l2"=w304:i32)  [unwired: 11 in]
      n150 = Index Array(array=w321, index #1=w287, index #2=w288, index #3=w289, index #4=w290, index #5=w291, index #6=w302, index #7=w292, index #8=w293, index #9=w294, index #10=w295, index #11=w296, index #12=w303, index #13=w297, index #14=w298, index #15=w299, index #16=w300, index #17=w301, index #18=w304) -> (element #1=w393:u16, element #2=w392:u16, element #3=w391:u16, element #4=w390:u16, element #5=w389:u16, element #6=w388:u16, element #7=w387:u16, element #8=w386:u16, element #9=w385:u16, element #10=w384:u16, element #11=w383:u16, element #12=w382:u16, element #13=w381:u16, element #14=w380:u16, element #15=w379:u16, element #16=w378:u16, element #17=w377:u16, element #18=w376:u16)
      n151 = Not Equal To 0?(x=w393) -> (x != 0?=w399:bool)
      n152 = Not Equal To 0?(x=w389) -> (x != 0?=w398:bool)
      n153 = Not Equal To 0?(x=w387) -> (x != 0?=w397:bool)
      n154 = Not Equal To 0?(x=w383) -> (x != 0?=w396:bool)
      n155 = Not Equal To 0?(x=w381) -> (x != 0?=w395:bool)
      n156 = Not Equal To 0?(x=w377) -> (x != 0?=w394:bool)
      n157 = local write "LC_ENL_First_OnOff"(w399) -> ()
      n158 = local write "LC_ENL_First_Block"(w392) -> ()
      n159 = local write "LC_ENL_First_Probability"(w391) -> ()
      n160 = local write "LC_ENL_First_Tdelay"(w390) -> ()
      n161 = local write "LC_ENL_First_delayOpt"(w398) -> ()
      n162 = local write "LC_ENL_First_Count"(w388) -> ()
      n163 = local write "LC_ENL_PreR_OnOff"(w397) -> ()
      n164 = local write "LC_ENL_PreR_Block"(w386) -> ()
      n165 = local write "LC_ENL_PreR_Probability"(w385) -> ()
      n166 = local write "LC_ENL_PreR_Tdelay"(w384) -> ()
      n167 = local write "LC_ENL_PreR_delayOpt"(w396) -> ()
      n168 = local write "LC_ENL_PreR_Count"(w382) -> ()
      n169 = local write "LC_ENL_PostR_OnOff"(w395) -> ()
      n170 = local write "LC_ENL_PostR_Block"(w380) -> ()
      n171 = local write "LC_ENL_PostR_Probability"(w379) -> ()
      n172 = local write "LC_ENL_PostR_Tdelay"(w378) -> ()
      n173 = local write "LC_ENL_PostR_delayOpt"(w394) -> ()
      n174 = local write "LC_ENL_PostR_Count"(w376) -> ()
      n175 = call "BRig_dataLC_Cue_First_OnOff_l2.vi"() -> ("output_Cue_First_OnOff_l2"=w281:i32)  [unwired: 11 in]
      n176 = call "BRig_dataLC_Cue_First_Block_l2.vi"() -> ("output_Cue_First_Block_l2"=w282:i32)  [unwired: 11 in]
      n177 = call "BRig_dataLC_Cue_First_Prob_l2.vi"() -> ("output_Cue_First_Prob_l2"=w283:i32)  [unwired: 11 in]
      n178 = call "BRig_dataLC_Cue_First_Delay_l2.vi"() -> ("output_Cue_First_Delay_l2"=w284:i32)  [unwired: 11 in]
      n179 = call "BRig_dataLC_Cue_First_DelayOpt_l2.vi"() -> ("output_Cue_First_DelayOpt_l2"=w285:i32)  [unwired: 11 in]
      n180 = call "BRig_dataLC_Cue_First_Count_l2.vi"() -> ("output_Cue_First_Count_l2"=w286:i32)  [unwired: 11 in]
      n181 = call "BRig_dataLC_Cue_PreR_OnOff_l2.vi"() -> ("output_Cue_PreR_OnOff_l2"=w246:i32)  [unwired: 11 in]
      n182 = call "BRig_dataLC_Cue_PreR_Block_l2.vi"() -> ("output_Cue_PreR_Block_l2"=w245:i32)  [unwired: 11 in]
      n183 = call "BRig_dataLC_Cue_PreR_Prob_l2.vi"() -> ("output_Cue_PreR_Prob_l2"=w244:i32)  [unwired: 11 in]
      n184 = call "BRig_dataLC_Cue_PreR_Delay_l2.vi"() -> ("output_Cue_PreR_Delay_l2"=w243:i32)  [unwired: 11 in]
      n185 = call "BRig_dataLC_Cue_PreR_DelayOpt_l2.vi"() -> ("output_Cue_PreR_DelayOpt_l2"=w242:i32)  [unwired: 11 in]
      n186 = call "BRig_dataLC_Cue_PreR_Count_l2.vi"() -> ("output_Cue_PreR_Count_l2"=w247:i32)  [unwired: 11 in]
      n187 = call "BRig_dataLC_Cue_PostR_OnOff_l2.vi"() -> ("output_Cue_PostR_OnOff_l2"=w240:i32)  [unwired: 11 in]
      n188 = call "BRig_dataLC_Cue_PostR_Block_l2.vi"() -> ("output_Cue_PostR_Block_l2"=w239:i32)  [unwired: 11 in]
      n189 = call "BRig_dataLC_Cue_PostR_Prob_l2.vi"() -> ("output_Cue_PostR_Prob_l2"=w238:i32)  [unwired: 11 in]
      n190 = call "BRig_dataLC_Cue_PostR_Delay_l2.vi"() -> ("output_Cue_PostR_Delay_l2"=w237:i32)  [unwired: 11 in]
      n191 = call "BRig_dataLC_Cue_PostR_DelayOpt_l2.vi"() -> ("output_Cue_PostR_DelayOpt_l2"=w236:i32)  [unwired: 11 in]
      n192 = call "BRig_dataLC_Cue_PostR_Count_l2.vi"() -> ("output_Cue_PostR_Count_l2"=w241:i32)  [unwired: 11 in]
      n193 = call "BRig_dataExp_LED_baseline_l2.vi"() -> ("output_LED_baseline_l2"=w258:i32)  [unwired: 11 in]
      n194 = call "BRig_dataExp_L_freq_l2.vi"() -> ("output_L_freq_l2"=w259:i32)  [unwired: 11 in]
      n195 = call "BRig_dataExp_L_T_l2.vi"() -> ("output_L_T_l2"=w260:i32)  [unwired: 11 in]
      n196 = call "BRig_dataExp_L_Tpeak_l2.vi"() -> ("output_L_Tpeak_l2"=w261:i32)  [unwired: 11 in]
      n197 = call "BRig_dataExp_L_Tshutter_l2.vi"() -> ("output_L_Tshutter_l2"=w262:i32)  [unwired: 11 in]
      n198 = call "BRig_dataExp_L_power_min_l2.vi"() -> ("output_L_power_min_l2"=w263:i32)  [unwired: 11 in]
      n199 = call "BRig_dataExp_L_power_max_l2.vi"() -> ("output_L_power_max_l2"=w264:i32)  [unwired: 11 in]
      n200 = call "BRig_dataExp_L_power_step_l2.vi"() -> ("output_L_power_step_l2"=w265:i32)  [unwired: 11 in]
      n201 = Index Array(array=w321, index #1=w281, index #2=w282, index #3=w283, index #4=w284, index #5=w285, index #6=w286, index #7=w246, index #8=w245, index #9=w244, index #10=w243, index #11=w242, index #12=w247, index #13=w240, index #14=w239, index #15=w238, index #16=w237, index #17=w236, index #18=w241) -> (element #1=w369:u16, element #2=w368:u16, element #3=w367:u16, element #4=w366:u16, element #5=w365:u16, element #6=w364:u16, element #7=w363:u16, element #8=w362:u16, element #9=w361:u16, element #10=w360:u16, element #11=w359:u16, element #12=w358:u16, element #13=w357:u16, element #14=w356:u16, element #15=w355:u16, element #16=w354:u16, element #17=w353:u16, element #18=w352:u16)
      n202 = Index Array(array=w235, index #1=w258, index #2=w259, index #3=w260, index #4=w261, index #5=w262, index #6=w263, index #7=w264, index #8=w265) -> (element #1=w320:u16, element #2=w318:u16, element #3=w317:u16, element #4=w316:u16, element #5=w315:u16, element #6=w314:u16, element #7=w313:u16, element #8=w312:u16)
      n203 = To Double Precision Float(number=w314) -> (double precision float=w311:dbl)
      n204 = To Double Precision Float(number=w313) -> (double precision float=w306:dbl)
      n205 = To Double Precision Float(number=w312) -> (double precision float=w305:dbl)
      n206 = Not Equal To 0?(x=w369) -> (x != 0?=w375:bool)
      n207 = Not Equal To 0?(x=w365) -> (x != 0?=w374:bool)
      n208 = Not Equal To 0?(x=w363) -> (x != 0?=w373:bool)
      n209 = Not Equal To 0?(x=w359) -> (x != 0?=w372:bool)
      n210 = Not Equal To 0?(x=w357) -> (x != 0?=w371:bool)
      n211 = Not Equal To 0?(x=w353) -> (x != 0?=w370:bool)
      n212 = Divide(x=w311, y=w307) -> (x/y=w310:dbl)
      n213 = Divide(x=w306, y=w307) -> (x/y=w309:dbl)
      n214 = Divide(x=w305, y=w307) -> (x/y=w308:dbl)
      n215 = local write "LC_Cue_First_OnOff"(w375) -> ()
      n216 = local write "LC_Cue_First_Block"(w368) -> ()
      n217 = local write "LC_Cue_First_Probability"(w367) -> ()
      n218 = local write "LC_Cue_First_Tdelay"(w366) -> ()
      n219 = local write "LC_Cue_First_delayOpt"(w374) -> ()
      n220 = local write "LC_Cue_First_Count"(w364) -> ()
      n221 = local write "LC_Cue_PreR_OnOff"(w373) -> ()
      n222 = local write "LC_Cue_PreR_Block"(w362) -> ()
      n223 = local write "LC_Cue_PreR_Probability"(w361) -> ()
      n224 = local write "LC_Cue_PreR_Tdelay"(w360) -> ()
      n225 = local write "LC_Cue_PreR_delayOpt"(w372) -> ()
      n226 = local write "LC_Cue_PreR_Count"(w358) -> ()
      n227 = local write "LC_Cue_PostR_OnOff"(w371) -> ()
      n228 = local write "LC_Cue_PostR_Block"(w356) -> ()
      n229 = local write "LC_Cue_PostR_Probability"(w355) -> ()
      n230 = local write "LC_Cue_PostR_Tdelay"(w354) -> ()
      n231 = local write "LC_Cue_PostR_delayOpt"(w370) -> ()
      n232 = local write "LC_Cue_PostR_Count"(w352) -> ()
      n233 = Not Equal To 0?(x=w320) -> (x != 0?=w319:bool)
      n234 = local write "LED_baseline"(w319) -> ()
      n235 = local write "Laser_Freq"(w318) -> ()
      n236 = local write "Laser_T"(w317) -> ()
      n237 = local write "Laser_Tpeak"(w316) -> ()
      n238 = local write "Laser_Tshutter"(w315) -> ()
      n239 = local write "Laser_power_min"(w310) -> ()
      n240 = local write "Laser_power_max"(w309) -> ()
      n241 = local write "Laser_power_step"(w308) -> ()
      n242 = call "BRig_dataLC_Selection_First_OnOff_l2.vi"() -> ("output_Selection_First_OnOff_l2"=w266:i32)  [unwired: 11 in]
      n243 = call "BRig_dataLC_Selection_First_Block_l2.vi"() -> ("output_Selection_First_Block_l2"=w267:i32)  [unwired: 11 in]
      n244 = call "BRig_dataLC_Selection_First_Prob_l2.vi"() -> ("output_Selection_First_Prob_l2"=w268:i32)  [unwired: 11 in]
      n245 = call "BRig_dataLC_Selection_First_Delay_l2.vi"() -> ("output_Selection_First_Delay_l2"=w269:i32)  [unwired: 11 in]
      n246 = call "BRig_dataLC_Selection_First_Count_l2.vi"() -> ("output_Selection_First_Count_l2"=w278:i32)  [unwired: 11 in]
      n247 = call "BRig_dataLC_Selection_PreR_OnOff_l2.vi"() -> ("output_Selection_PreR_OnOff_l2"=w270:i32)  [unwired: 11 in]
      n248 = call "BRig_dataLC_Selection_PreR_Block_l2.vi"() -> ("output_Selection_PreR_Block_l2"=w271:i32)  [unwired: 11 in]
      n249 = call "BRig_dataLC_Selection_PreR_Prob_l2.vi"() -> ("output_Selection_PreR_Prob_l2"=w272:i32)  [unwired: 11 in]
      n250 = call "BRig_dataLC_Selection_PreR_Delay_l2.vi"() -> ("output_Selection_PreR_Delay_l2"=w273:i32)  [unwired: 11 in]
      n251 = call "BRig_dataLC_Selection_PreR_Count_l2.vi"() -> ("output_Selection_PreR_Count_l2"=w279:i32)  [unwired: 11 in]
      n252 = call "BRig_dataLC_Selection_PostR_OnOff_l2.vi"() -> ("output_Selection_PostR_OnOff_l2"=w274:i32)  [unwired: 11 in]
      n253 = call "BRig_dataLC_Selection_PostR_Block_l2.vi"() -> ("output_Selection_PostR_Block_l2"=w275:i32)  [unwired: 11 in]
      n254 = call "BRig_dataLC_Selection_PostR_Prob_l2.vi"() -> ("output_Selection_PostR_Prob_l2"=w276:i32)  [unwired: 11 in]
      n255 = call "BRig_dataLC_Selection_PostR_Delay_l2.vi"() -> ("output_Selection_PostR_Delay_l2"=w277:i32)  [unwired: 11 in]
      n256 = call "BRig_dataLC_Selection_PostR_Count_l2.vi"() -> ("output_Selection_PostR_Count_l2"=w280:i32)  [unwired: 11 in]
      n257 = call "BRig_dataLC_Reward_OnOff_l2.vi"() -> ("output_Reward_OnOff_l2"=w248:i32)  [unwired: 11 in]
      n258 = call "BRig_dataLC_Reward_Block_l2.vi"() -> ("output_Reward_Block_l2"=w249:i32)  [unwired: 11 in]
      n259 = call "BRig_dataLC_Reward_Trial_l2.vi"() -> ("output_Reward_Trial_l2"=w250:i32)  [unwired: 11 in]
      n260 = call "BRig_dataLC_Reward_Prob_l2.vi"() -> ("output_Reward_Prob_l2"=w251:i32)  [unwired: 11 in]
      n261 = call "BRig_dataLC_Reward_Delay_l2.vi"() -> ("output_Reward_Delay_l2"=w256:i32)  [unwired: 11 in]
      n262 = call "BRig_dataLC_Wrong_OnOff_l2.vi"() -> ("output_Wrong_OnOff_l2"=w252:i32)  [unwired: 11 in]
      n263 = call "BRig_dataLC_Wrong_Block_l2.vi"() -> ("output_Wrong_Block_l2"=w253:i32)  [unwired: 11 in]
      n264 = call "BRig_dataLC_Wrong_Trial_l2.vi"() -> ("output_Wrong_Trial_l2"=w254:i32)  [unwired: 11 in]
      n265 = call "BRig_dataLC_Wrong_Prob_l2.vi"() -> ("output_Wrong_Prob_l2"=w255:i32)  [unwired: 11 in]
      n266 = call "BRig_dataLC_Wrong_Delay_l2.vi"() -> ("output_Wrong_Delay_l2"=w257:i32)  [unwired: 11 in]
      n267 = Index Array(array=w321, index #1=w248, index #2=w249, index #3=w250, index #4=w251, index #5=w256, index #6=w252, index #7=w253, index #8=w254, index #9=w255, index #10=w257) -> (element #1=w331:u16, element #2=w330:u16, element #3=w329:u16, element #4=w328:u16, element #5=w327:u16, element #6=w326:u16, element #7=w325:u16, element #8=w324:u16, element #9=w323:u16, element #10=w322:u16)
      n268 = Index Array(array=w321, index #1=w266, index #2=w267, index #3=w268, index #4=w269, index #5=w278, index #6=w270, index #7=w271, index #8=w272, index #9=w273, index #10=w279, index #11=w274, index #12=w275, index #13=w276, index #14=w277, index #15=w280) -> (element #1=w348:u16, element #2=w347:u16, element #3=w346:u16, element #4=w345:u16, element #5=w344:u16, element #6=w343:u16, element #7=w342:u16, element #8=w341:u16, element #9=w340:u16, element #10=w339:u16, element #11=w338:u16, element #12=w337:u16, element #13=w336:u16, element #14=w335:u16, element #15=w334:u16)
      n269 = Not Equal To 0?(x=w331) -> (x != 0?=w333:bool)
      n270 = Not Equal To 0?(x=w326) -> (x != 0?=w332:bool)
      n271 = Not Equal To 0?(x=w348) -> (x != 0?=w351:bool)
      n272 = Not Equal To 0?(x=w343) -> (x != 0?=w350:bool)
      n273 = Not Equal To 0?(x=w338) -> (x != 0?=w349:bool)
      n274 = local write "LC_Reward_OnOff"(w333) -> ()
      n275 = local write "LC_Reward_Block"(w330) -> ()
      n276 = local write "LC_Reward_Trial"(w329) -> ()
      n277 = local write "LC_Reward_Probability"(w328) -> ()
      n278 = local write "LC_Reward_Tdelay"(w327) -> ()
      n279 = local write "LC_Wrong_OnOff"(w332) -> ()
      n280 = local write "LC_Wrong_Block"(w325) -> ()
      n281 = local write "LC_Wrong_Trial"(w324) -> ()
      n282 = local write "LC_Wrong_Probability"(w323) -> ()
      n283 = local write "LC_Wrong_Tdelay"(w322) -> ()
      n284 = local write "LC_Sel_First_OnOff"(w351) -> ()
      n285 = local write "LC_Sel_First_Block"(w347) -> ()
      n286 = local write "LC_Sel_First_Probability"(w346) -> ()
      n287 = local write "LC_Sel_First_Tdelay"(w345) -> ()
      n288 = local write "LC_Sel_First_Count"(w344) -> ()
      n289 = local write "LC_Sel_PreR_OnOff"(w350) -> ()
      n290 = local write "LC_Sel_PreR_Block"(w342) -> ()
      n291 = local write "LC_Sel_PreR_Probability"(w341) -> ()
      n292 = local write "LC_Sel_PreR_Tdelay"(w340) -> ()
      n293 = local write "LC_Sel_PreR_Count"(w339) -> ()
      n294 = local write "LC_Sel_PostR_OnOff"(w349) -> ()
      n295 = local write "LC_Sel_PostR_Block"(w337) -> ()
      n296 = local write "LC_Sel_PostR_Probability"(w336) -> ()
      n297 = local write "LC_Sel_PostR_Tdelay"(w335) -> ()
      n298 = local write "LC_Sel_PostR_Count"(w334) -> ()
    }
  }
  "output_dataLC" <- w4
  "output_dataExp" <- w1
